vi "Set_Bandwidth.vi"   [LabVIEW 2010, in "FEMTO_LUCI-10.lvlib"]
doc: "This function sets the bandwidth for the selected device."
uses:
  <userlib>/FEMTO/FEMTO_LUCI-10.lvlib
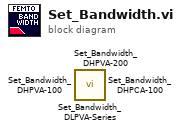
[diagram p0: block diagram]
diagram:
  n1 = call <userlib>:"Set_Bandwidth_DLPVA-Series.vi"() -> ()  [unwired: 4 in, 3 out]
  n2 = call <userlib>:"Set_Bandwidth_DHPVA-200.vi"() -> ()  [unwired: 4 in, 3 out]
  n3 = call <userlib>:"Set_Bandwidth_DHPVA-100.vi"() -> ()  [unwired: 4 in, 3 out]
  n4 = call <userlib>:"Set_Bandwidth_DHPCA-100.vi"() -> ()  [unwired: 4 in, 3 out]
